vi "DataTranslation_global.vi"() -> ()   [LabVIEW 2010]
panel:
  out "DT Task ID":i32
  in  "Different Sampling Freq per block":bool
  in  "Orifice Diameter (mm)":dbl=20.0
  out "Freqs":dbl[](array[numeric])
  out "Amps":dbl[](array[numeric])
  out "Amplitudes":dbl[](array[numeric])
  out "Frequencies":dbl[](array[numeric])
  in  "Dwell (ms)":u32=500
  out "Number of cycles":dbl=5.0
  in  "Samples per cycle":dbl=20.0
  in  "Device Name":refnum<visa-resource-name>="USB0::0x0699::0x0347::C036837::INSTR"
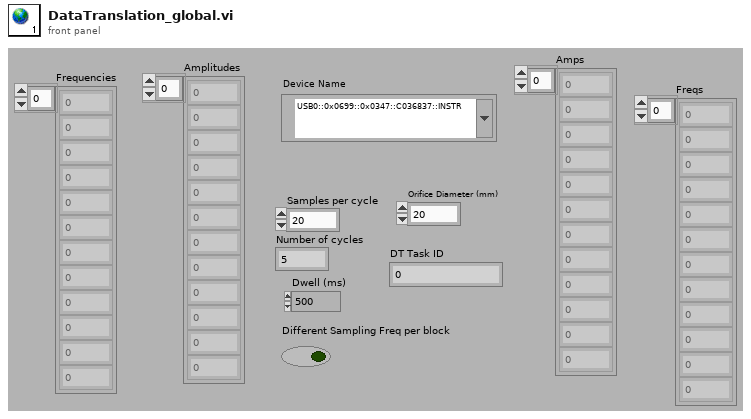
[diagram p1: front panel]
diagram:
